vi "RT - Process Acquire Loop Error Flags.vi"(8 "error in (no error)":errorcluster caption="错误输入（无错误）", 11 "Error Flags":bool[](array[boolean]) caption="错误标志") -> (0 "error out":errorcluster caption="错误输出")   [LabVIEW 2013]
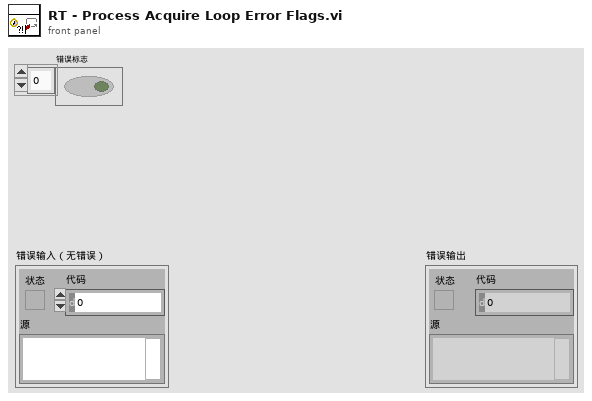
[diagram p1: front panel]
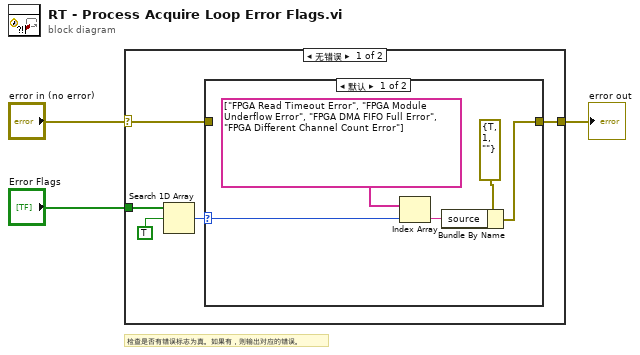
[diagram p0: block diagram]
diagram:
  # "检查是否有错误标志为真。如果有，则输出对应的错误。"
  n1 = case shown="无错误" "error in (no error)" {
    selector: "error in (no error)" -> [w5 w15]
    tunnel: [w4 w15] -> w2
    tunnel: "Error Flags" -> [w8 _]
    frame No Error {
      n2 = Search 1D Array(1D array=w8, element=TRUE) -> (index of element=w6:i32)  [unwired: 1 in]
      n3 = case shown="默认" w6 {
        selector: w6 -> [w11 _]
        tunnel: w5 -> [_ w14]
        tunnel: [w12 w14] -> w4
        frame Default {
          n4 = Index Array(array=string[] ["FPGA Read Timeout Error", "FPGA Module Underflow Error", "FPGA DMA FIFO Full Error", "FPGA Different Channel Count Error"], index=w11) -> (element=w10:string)
          n5 = Bundle By Name(cluster=errorcluster {"status"=TRUE, "code"=1, "source"=""} ("error constant"), "source"=w10) -> (w12:errorcluster)
        }
        frame -1 {
        }
      }
    }
    frame Error {
    }
  }
  "error out" <- w2
